vi "niRFUtil CONV DBL to Coerced DBL.vi"(6 "Error Limit":dbl=1e-10 format="%#.16g", 11 "Numeric In (DBL)":dbl format="%#.16g") -> (3 "Coerced Numeric Out (DBL)":dbl format="%#.16g")   [LabVIEW 2016, in "niRFUtil.lvlib"]
doc: "This VI is used to remove the small fractions (of the order of E-12) that are present in the floating point representation of a number."
uses:
  niRFUtil.lvlib
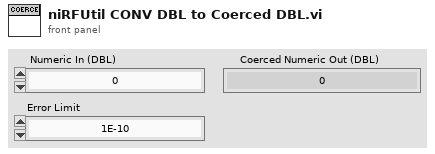
[diagram p1: front panel]
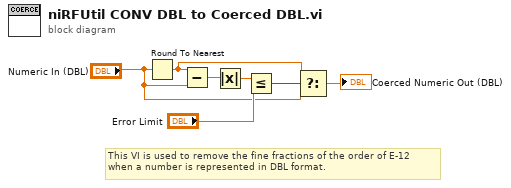
[diagram p0: block diagram]
diagram:
  # "This VI is used to remove the fine fractions of the order of E-12 \nwhen a number is represented in DBL format."
  n1 = Round To Nearest(number="Numeric In (DBL)") -> (nearest integer value=w2:dbl)
  n2 = Subtract(x=w2, y="Numeric In (DBL)") -> (x-y=w6:dbl)
  n3 = Absolute Value(x=w6) -> (abs(x)=w5:dbl)
  n4 = Less Or Equal?(x=w5, y="Error Limit") -> (x <= y?=w3:bool)
  n5 = Select(t=w2, s=w3, f="Numeric In (DBL)") -> (s? t:f=→"Coerced Numeric Out (DBL)":dbl)
